vi "main.vi"() -> ()   [LabVIEW 2014]
panel:
  in  "采集数据":bool
  out "D3":sgl
  in  "出口温度(D8)":i16(knob) scale=0.0..100.0
  in  "D9":i16(slide) scale=-100.0..100.0
  out "D2":dbl
  out "D1":dbl
  out "通讯失败":string="三菱PLC通讯失败，串口已关闭！"
  in  "打开串口":bool
  out "温度曲线":cluster{sgl, sgl}(graph)
  in  "进口温度(D7)":i16(knob) scale=0.0..100.0
  in  "Y11":bool
  in  "Y1":bool
  in  "Y17":bool
  in  "Y16":bool
  in  "Y15":bool
  in  "Y14":bool
  in  "Y13":bool
  in  "Y12":bool
  in  "Y10":bool
  in  "Y7":bool
  in  "Y6":bool
  in  "Y5":bool
  in  "Y4":bool
  in  "Y3":bool
  in  "Y2":bool
  in  "Y0":bool
  out "X11":bool
  out "X1":bool
  out "X17":bool
  out "X16":bool
  out "X15":bool
  out "X14":bool
  out "X13":bool
  out "X12":bool
  out "X10":bool
  out "X7":bool
  out "X6":bool
  out "X5":bool
  out "X4":bool
  out "X3":bool
  out "X2":bool
  out "X0":bool
  out "EXIT":bool
  # "输入监控指示"
  # "输出控制"
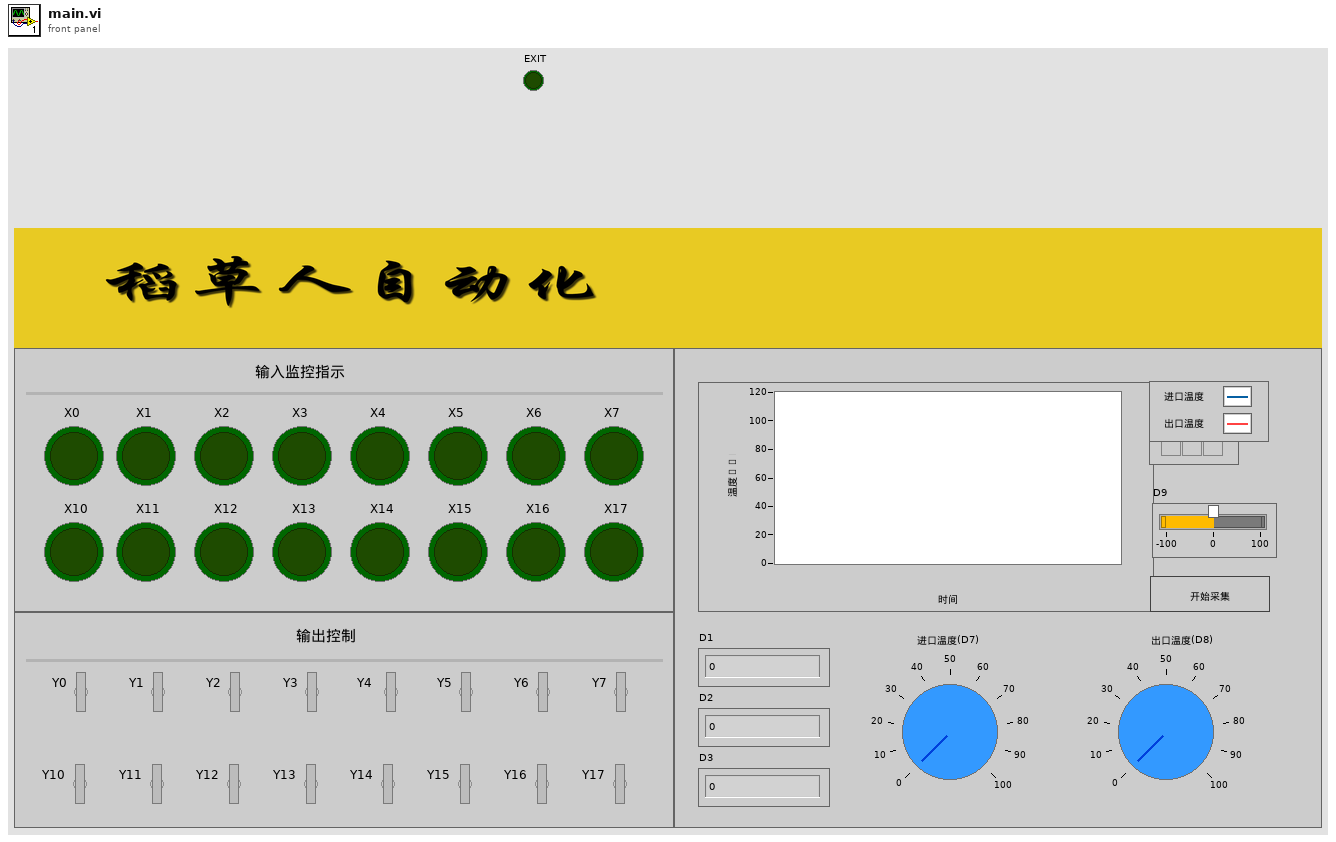
[diagram p1: front panel]
types:
  T1 = enum16{"open", "replace", "create", "open or create", "replace or create", "replace or create with confirmation"}
  T2 = cluster{"通讯串口":refnum<visa-resource-name>, "波特率":u32, "数据比特":u16, "奇偶校验":enum16{"None", "Odd", "Even", "Mark", "Space"}, "停止位":u16, "等待延时(ms)":u32}
  T3 = enum16{"open", "open or create", "create or replace", "create", "open (read-only)"}
  T4 = enum32{"invalid app kind", "Development System", "Run Time System", "Student Edition", "Embedded LabVIEW", "Evaluation", "Custom"}
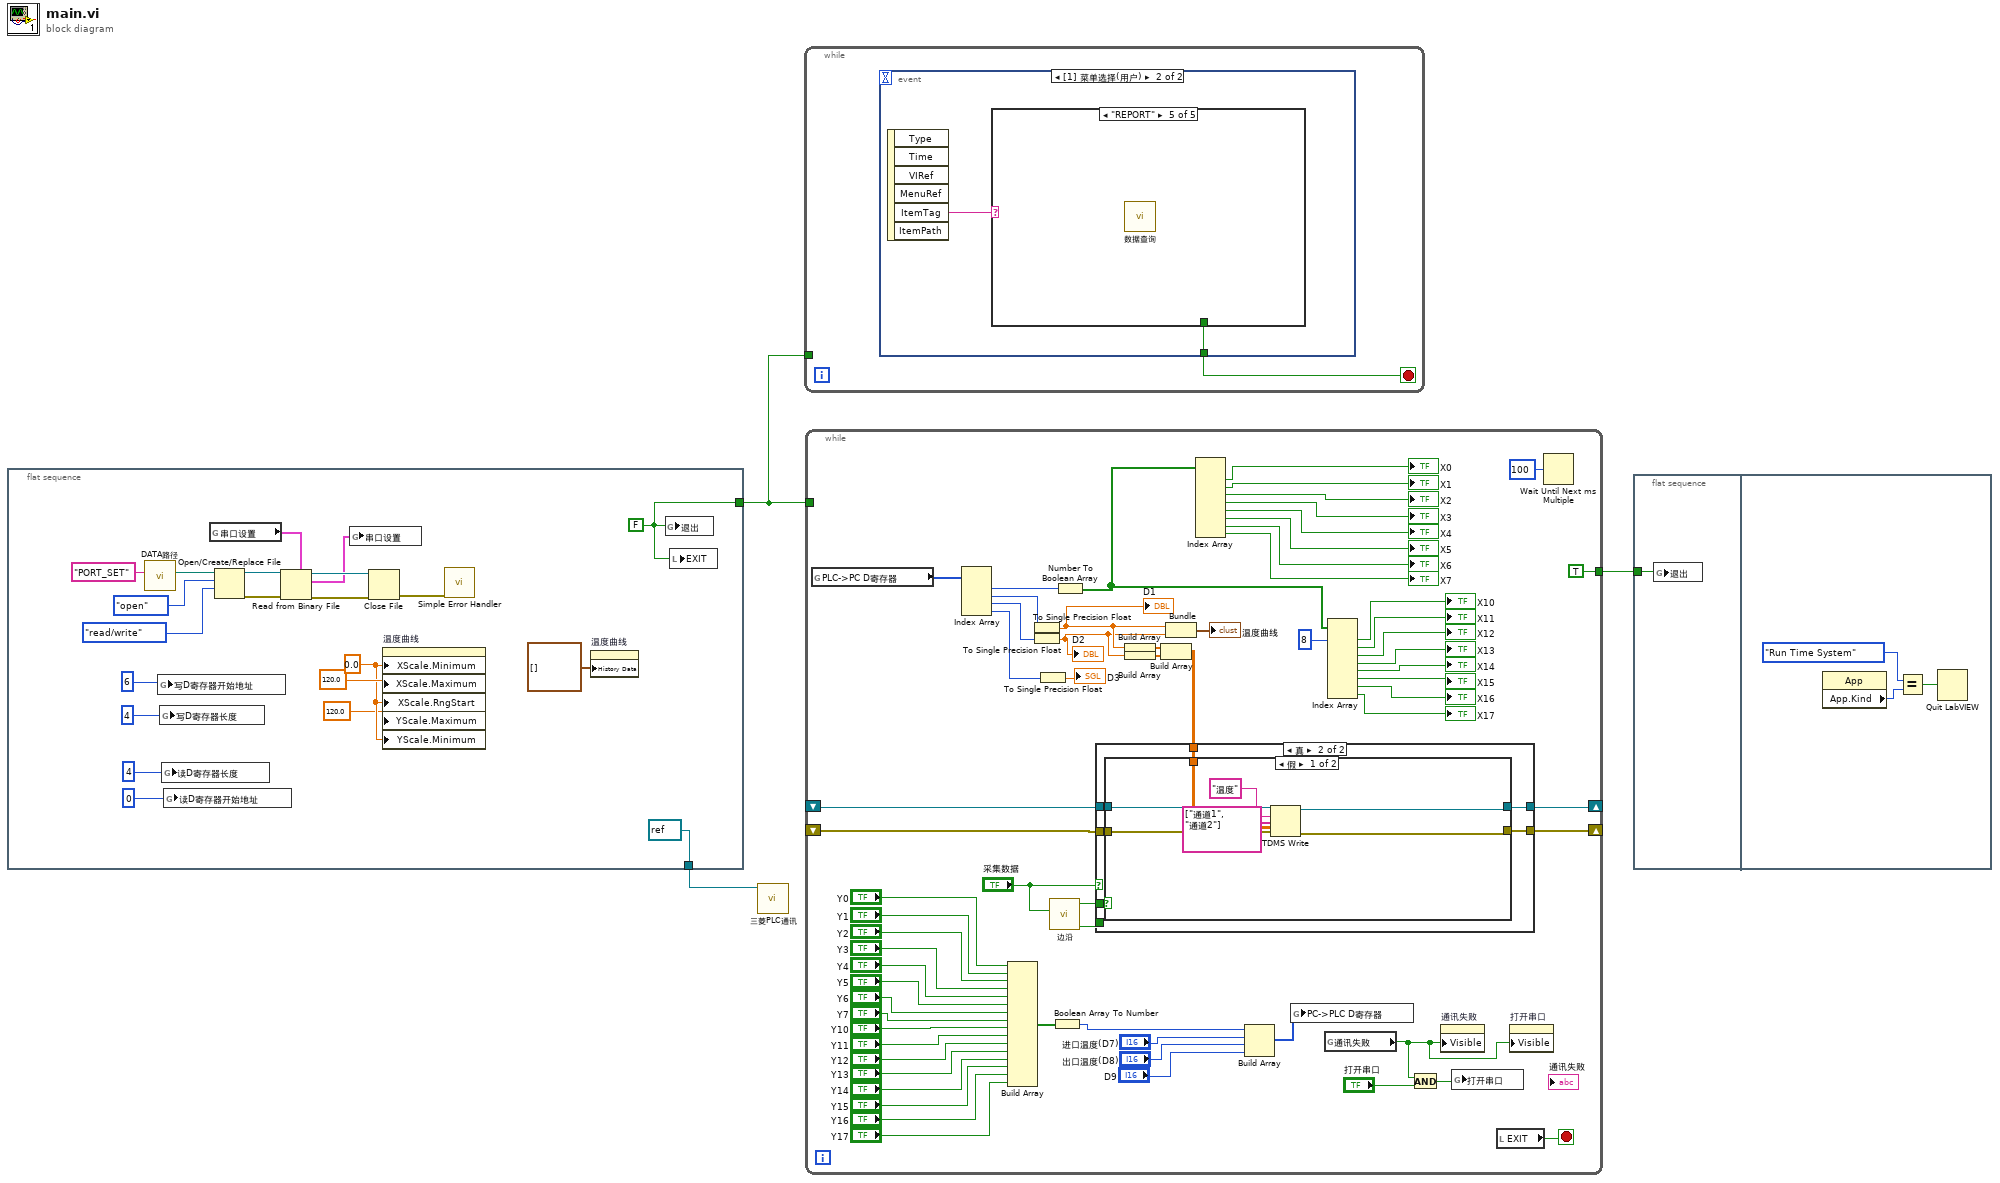
[diagram p0: block diagram]
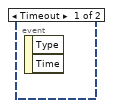
[diagram p2: hidden frame]
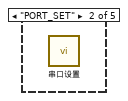
[diagram p4: hidden frame]
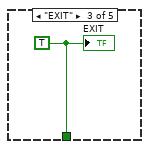
[diagram p5: hidden frame]
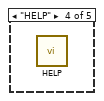
[diagram p6: hidden frame]
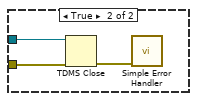
[diagram p8: hidden frame]
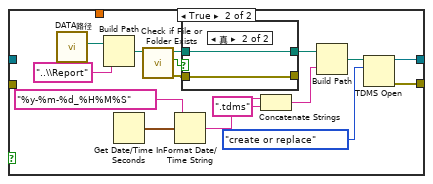
[diagram p9: hidden frame]
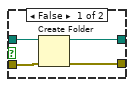
[diagram p10: hidden frame]
diagram:
  n1 = flat-sequence {
    tunnel: [w24] -> w2
    tunnel: [refnum<visa-resource-name> refnum ("VISA resource name")] -> w1
    frame #0 {
      w6 = 0.0 ("X标尺.范围:最大值")
      w24 = FALSE ("退出")
      n2 = call "DATA路径.vi"("文件名"="PORT_SET") -> ("DATA路径"=w11:path)  [unwired: 10 in]
      n3 = global write "三菱全局变量.vi" "写D寄存器开始地址"(u16 6 ("写D寄存器开始地址")) -> ()
      n4 = global write "三菱全局变量.vi" "写D寄存器长度"(u16 4 ("写D寄存器长度")) -> ()
      n5 = global write "三菱全局变量.vi" "读D寄存器长度"(u16 4 ("写D寄存器开始地址")) -> ()
      n6 = global write "三菱全局变量.vi" "读D寄存器开始地址"(u16 0 ("读D寄存器开始地址")) -> ()
      n7 = global read "三菱全局变量.vi" "串口设置"() -> (w10:T2)
      n8 = Open/Create/Replace File(file path (use dialog)=w11, operation (0:open)=T1."open" ("操作(0:open)"), access (0:read/write)=enum16{"read/write", "read-only", "write-only"}."read/write" ("权限(0:read/write)")) -> (refnum out=w16:refnum<file>, error out=w15:errorcluster)  [unwired: 3 in, 1 out]
      n9 = Read from Binary File(5:w10, 8:w15, 11:w16) -> (0:w13:errorcluster, 2:w9:T2, 3:w14:refnum<file>)  [unwired: 3 in, 1 out]
      n10 = global write "三菱全局变量.vi" "串口设置"(w9) -> ()
      n11 = Close File(refnum=w14, error in=w13) -> (error out=w12:errorcluster)  [unwired: 1 out]
      n12 = property on="温度曲线" class="WFChart (严格)"("XScale.Minimum"=w6, "XScale.Maximum"=120.0 ("X标尺.范围:最大值"), "XScale.RngStart"=w6, "YScale.Maximum"=120.0 ("Y标尺.范围:最大值"), "YScale.Minimum"=w6) -> ()  [unwired: 2 in, 2 out]
      n13 = call <vilib>:"Simple Error Handler.vi"("error in (no error)"=w12) -> ()  [unwired: 4 in, 5 out]
      n14 = property on="温度曲线" class="WFChart (严格)"("History Data"=cluster{sgl, sgl}[] [] ("历史数据")) -> ()  [unwired: 2 in, 2 out]
      n15 = global write "三菱全局变量.vi" "退出"(w24) -> ()
      n16 = local write "EXIT"(w24) -> ()
    }
  }
  n17 = call "三菱PLC通讯.vi"("VISA resource name"=w1) -> ()  [unwired: 11 in]
  n18 = while {
    tunnel: w2 -> [_]
    stop <- w25 stop-if-true
    n19 = event shown="[1] 菜单选择(用户)" {
      selector: _ -> [_ _]
      dyn-events: _ -> [_ _]
      timeout: _ -> [_ _]
      tunnel: [_ w26] -> w25
      event Timeout {
        n20 = event-data() -> ()  [unwired: 1 in, 2 out]
      }
      event Menu Selection (User) {
        n21 = event-data() -> ("ItemTag"=w27:string)  [unwired: 1 in, 5 out]
        n22 = case shown="\"REPORT\"" w27 {
          tunnel: [_ _ w28 _ _] -> w26
          frame "TRUE", Default {
          }
          frame "PORT_SET" {
            n23 = call "串口设置.vi"() -> ()  [unwired: 12 in]
          }
          frame "EXIT" {
            w28 = TRUE ("EXIT")
            "EXIT" <- w28
          }
          frame "HELP" {
            n24 = call "HELP.vi"() -> ()  [unwired: 12 in]
          }
          frame "REPORT" {
            n25 = call "数据查询.vi"() -> ()  [unwired: 12 in]
          }
        }
      }
    }
  }
  n26 = while {
    tunnel: w2 -> [_]
    tunnel: [TRUE ("退出")] -> w3
    shift-right: [w39] -> _
    shift-left: _ -> [w37]
    shift-right: [w38] -> _
    shift-left: _ -> [w36]
    stop <- w93 stop-if-true
    n27 = global read "三菱全局变量.vi" "PLC->PC D寄存器"() -> (w91:i16[])
    n28 = Index Array(array=w91) -> (element #1=w87:i16, element #2=w86:i16, element #3=w85:i16, element #4=w65:i16)  [unwired: 4 in]
    n29 = Build Array("Y0", "Y1", "Y2", "Y3", "Y4", "Y5", "Y6", "Y7", "Y10", "Y11", "Y12", "Y13", "Y14", "Y15", "Y16", "Y17") -> (w48:bool[])
    n30 = To Single Precision Float(number=w86) -> (single precision float=w31:sgl)
    "D1" <- w31
    n31 = To Single Precision Float(number=w85) -> (single precision float=w29:sgl)
    "D2" <- w29
    n32 = To Single Precision Float(number=w65) -> (single precision float=→"D3":sgl)
    n33 = call "边沿.vi"("IN"="采集数据") -> ("下降沿"=w33:bool, "上升沿"=w40:bool)  [unwired: 9 in]
    n34 = Boolean Array To Number(Boolean array=w48) -> (number=w47:u32)
    n35 = Number To Boolean Array(number=w87) -> (Boolean array=w76:bool[])
    n36 = Build Array(w31) -> (w32:sgl[])
    n37 = Build Array(w29) -> (w30:sgl[])
    n38 = Build Array(w32, w30) -> (w34:sgl[][])
    n39 = case shown="真" "采集数据" {
      tunnel: w40 -> [_ w109]
      tunnel: [w95 w108] -> w39
      tunnel: [w94 w107] -> w38
      tunnel: w37 -> [w96 w106]
      tunnel: w36 -> [w97 w105]
      tunnel: w34 -> [_ w104]
      tunnel: w33 -> [w98 _]
      frame False {
        n40 = case shown="假" w98 {
          tunnel: w97 -> [w99 w103]
          tunnel: w96 -> [w100 w102]
          tunnel: [w100 _] -> w95
          tunnel: [w99 _] -> w94
          frame False {
          }
          frame True {
            n41 = TDMS Close(8:w103, 11:w102) -> (0:w101:errorcluster)  [unwired: 1 out]
            n42 = call <vilib>:"Simple Error Handler.vi"("error in (no error)"=w101) -> ()  [unwired: 4 in, 5 out]
          }
        }
      }
      frame True {
        n43 = case shown="假" w109 {
          tunnel: [w112 w118] -> w108
          tunnel: [w111 w117] -> w107
          tunnel: w106 -> [w116 _]
          tunnel: w105 -> [w115 _]
          tunnel: w104 -> [w113 _]
          frame False {
            n44 = TDMS Write(0:w116, 5:"温度" ("组名称输入（无标题）"), 7:string[] ["通道1", "通道2"] ("通道名输入（无标题）"), 9:w113, 11:w115) -> (4:w112:refnum<k34>, 15:w111:errorcluster)  [unwired: 1 in, 2 out]
          }
          frame True {
            n45 = call "DATA路径.vi"() -> ("DATA路径"=w132:path)  [unwired: 11 in]
            n46 = Build Path(base path=w132, name or relative path="..\\Report" ("名称或相对路径")) -> (appended path=w130:path)
            n47 = Get Date/Time In Seconds() -> (seconds since 1Jan1904=w124:timestamp)
            n48 = call <vilib>:"Check if File or Folder Exists.vi"("path"=w130) -> ("error out"=w127:errorcluster, "file or folder exists?"=w129:bool, "dup path"=w128:path)  [unwired: 8 in]
            n49 = Format Date/Time String(time format string (%c)="%y-%m-%d_%H%M%S" ("时间格式字符串(%c)"), seconds (now)=w124) -> (date/time string=w123:string)  [unwired: 1 in]
            n50 = case shown="真" w129 {
              tunnel: w128 -> [w136 w138]
              tunnel: w127 -> [w135 w137]
              tunnel: [w134 w138] -> w126
              tunnel: [w133 w137] -> _
              frame False {
                n51 = Create Folder(path (use dialog)=w136, error in=w135) -> (created path=w134:path, error out=w133:errorcluster)  [unwired: 1 in, 1 out]
              }
              frame True {
              }
            }
            n52 = Concatenate Strings(w123, ".tdms" ("字符串")) -> (w121:string)
            n53 = Build Path(base path=w126, name or relative path=w121) -> (appended path=w120:path)
            n54 = TDMS Open(10:T3."create or replace" ("操作(0:open)"), 11:w120) -> (0:w117:errorcluster, 3:w118:refnum<k34>)  [unwired: 5 in]
          }
        }
      }
    }
    n55 = Bundle(w31, w29) -> (→"温度曲线":cluster{sgl, sgl})  [unwired: 1 in]
    n56 = Index Array(array=w76) -> (element #1=→"X0":bool, element #2=→"X1":bool, element #3=→"X2":bool, element #4=→"X3":bool, element #5=→"X4":bool, element #6=→"X5":bool, element #7=→"X6":bool, element #8=→"X7":bool)  [unwired: 8 in]
    n57 = Build Array(w47, "进口温度(D7)", "出口温度(D8)", "D9") -> (w46:u32[])
    n58 = global write "三菱全局变量.vi" "PC->PLC D寄存器"(w46) -> ()
    n59 = global read "三菱全局变量.vi" "通讯失败"() -> (w89:bool)
    n60 = Index Array(array=w76, index #1=8 ("索引")) -> (element #1=→"X10":bool, element #2=→"X11":bool, element #3=→"X12":bool, element #4=→"X13":bool, element #5=→"X14":bool, element #6=→"X15":bool, element #7=→"X16":bool, element #8=→"X17":bool)  [unwired: 7 in]
    n61 = And(x=w89, y="打开串口") -> (x .and. y?=w90:bool)
    n62 = property on="通讯失败" class="Str"("Visible"=w89) -> ()  [unwired: 2 in, 2 out]
    n63 = global write "三菱全局变量.vi" "打开串口"(w90) -> ()
    n64 = local read "EXIT"() -> (w93:bool)
    n65 = property on="打开串口" class="Bool"("Visible"=w89) -> ()  [unwired: 2 in, 2 out]
    n66 = Wait Until Next ms Multiple(millisecond multiple=u32 100 ("毫秒倍数")) -> ()  [unwired: 1 out]
  }
  n67 = flat-sequence {
    tunnel: w3 -> [w139]
    frame #0 {
      n68 = global write "三菱全局变量.vi" "退出"(w139) -> ()
    }
    frame #1 {
      n69 = property class="App"() -> ("App.Kind"=w141:T4)  [unwired: 2 in, 2 out]
      n70 = Equal?(x=T4."Run Time System" ("应用程序:类别"), y=w141) -> (x = y?=w142:bool)
      n71 = Quit LabVIEW(quit? (T)=w142) -> ()
    }
  }
